vi "Read Independent Variables.vi"(8 "error in (no error)":errorcluster, 11 "Scanner.lvclass in":refnum<class "Scanner.lvclass">) -> (0 "error out":errorcluster, 1 "size":i32, 2 "Independent Variables":dbl[][](array[numeric]), 3 "Scanner.lvclass out":refnum<class "Scanner.lvclass">, 4 "min value":dbl, 5 "max value":dbl)   [LabVIEW 2017, in "Scanner.lvclass"]
doc: "Return the internal array of independent variables for this Scanner, e.g., to write out to a file. Use this method with extreme caution, since it breaks the encapsulation for this class. Do not use it to manipulate a Scanner's internal state."
uses:
  Scanner.lvclass
  Scanner.lvclass/Scanner.ctl
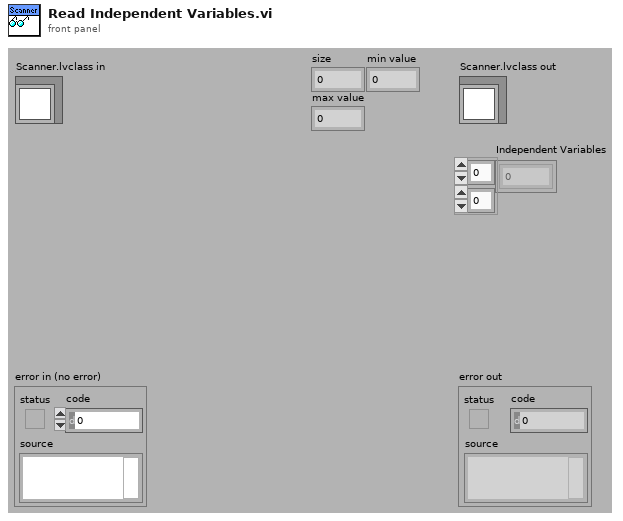
[diagram p1: front panel]
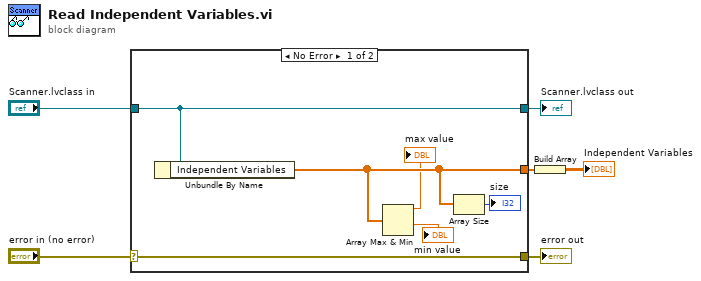
[diagram p0: block diagram]
diagram:
  n1 = case shown="No Error" "error in (no error)" {
    selector: "error in (no error)" -> [w12 w13]
    tunnel: [w12 w13] -> w5
    tunnel: [w11 w14] -> w3
    tunnel: "Scanner.lvclass in" -> [w11 w14]
    tunnel: [w9 _] -> w2
    frame No Error {
      n2 = Unbundle By Name(w11) -> ("Independent Variables"=w9:dbl[])
      n3 = Array Max & Min(array=w9) -> (max value=→"max value":dbl, min value=→"min value":dbl)  [unwired: 2 out]
      n4 = Array Size(array=w9) -> (size(s)=→"size":i32)
    }
    frame Error {
    }
  }
  "error out" <- w5
  "Scanner.lvclass out" <- w3
  n5 = Build Array(w2) -> (→"Independent Variables":dbl[][])
